vi "fn Write Item DBL.vi"(8 "error in (no error)":errorcluster, 10 "val":dbl, 11 "idx":i32) -> (0 "error out":errorcluster, 3 "idx out (dup)":i32)   [LabVIEW 2018, in "LV_OPC.lvlib"]
doc: "LVOPC_API int fnWriteItemDBL(int idx, double val);"
uses:
  LV_OPC.lvlib
  LVOPC64.dll
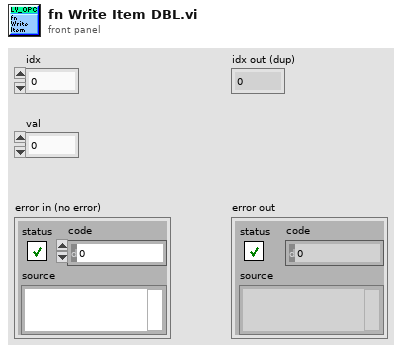
[diagram p1: front panel]
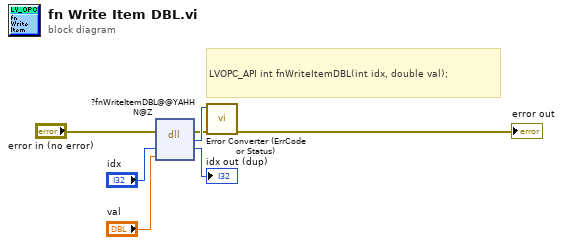
[diagram p0: block diagram]
diagram:
  # "LVOPC_API int fnWriteItemDBL(int idx, double val);"
  n1 = dll-call lib="C:/Users/Andrey/Desktop/LV_OPC-Client-x64/LV_OPC_Test/OPC.DLL/LVOPC64.*" fn="?fnWriteItemDBL@@YAHHN@Z"(error in="error in (no error)", "idx"="idx", "val"="val") -> (error out=w3:errorcluster, "return type"=w7:i32, "idx"=→"idx out (dup)":i32)  [unwired: 3 in, 1 out]
  n2 = call "Error Converter (ErrCode or Status).vi"("error in (no error)"=w3, "error code"=w7) -> ("error out"=→"error out":errorcluster)  [unwired: 9 in]
